vi "Game_Init.vi"(11 "display in":refnum<vi>) -> (0 "error out":errorcluster, 3 "class data out":refnum<class "Game.lvclass">)   [LabVIEW 2010, in "Labricks.lvlib" / "Game.lvclass"]
uses:
  Game.lvclass
  <vilib>/Utility/miscctls.llb/LV3DPointTypeDef.ctl
  BoundingBox_class/BoundingBox.lvclass
  RenderBase/SceneRoot_class/SceneRoot.lvclass
  Game.lvclass/Game.ctl
  Paddle_class/Paddle.lvclass
  Text_class/Text.lvclass
  Ball_class/Ball.lvclass
  RenderBase/SceneObject_class/properties/InitialPosition/SetInitialPosition.vi
  Ball_class/properties/InitialDirection/SetInitialDirection.vi
  RenderBase/Sprite_class/Sprite.lvclass
  RenderBase/SceneObject_class/SceneObject.lvclass
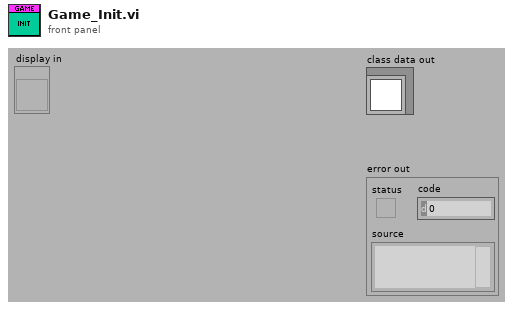
[diagram p1: front panel]
types:
  T1 = typedef "LV3DPointTypeDef.ctl" = cluster{"X":sgl, "Y":sgl, "Z":sgl}
  T2 = cluster{"X":sgl, "Y":sgl, "Width":sgl, "Height":sgl}
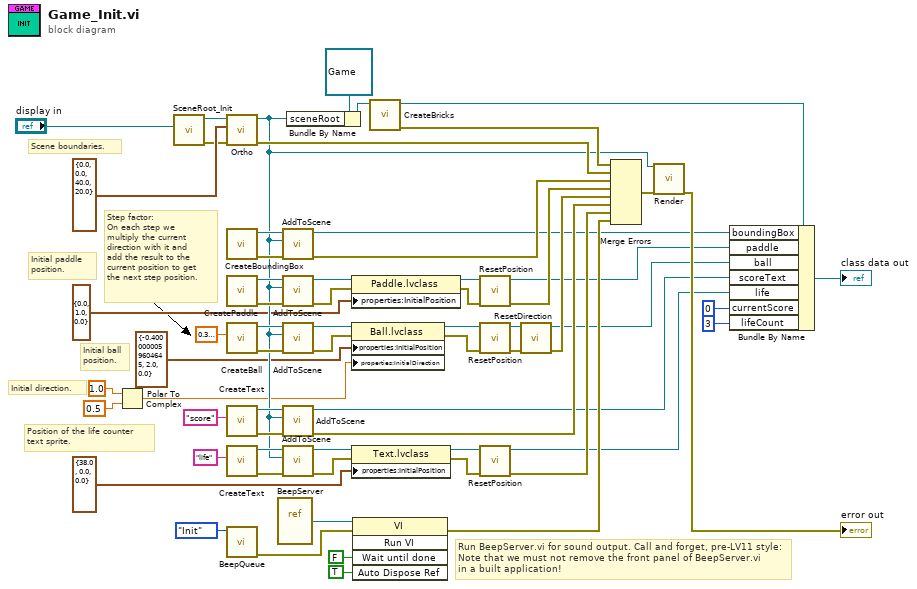
[diagram p0: block diagram]
diagram:
  # "Initial ball\nposition."
  # "Step factor:\nOn each step we\nmultiply the current\ndirection with it and\nadd the result to the\ncurrent position to get\nthe next step position."
  # "Position of the life counter\ntext sprite."
  # "Initial direction."
  # "Initial paddle \nposition."
  # "Scene boundaries."
  # "Run BeepServer.vi for sound output. Call and forget, pre-LV11 style:\nNote that we must not remove the front panel of BeepServer.vi\nin a built application!"
  n1 = Polar To Complex(1:sgl 0.5, 2:sgl 1.0 ("r")) -> (0:w9:csg)
  n2 = call "SceneRoot_Init.vi"("display in"="display in") -> ("error out"=w49:errorcluster, "class data out"=w59:refnum<class "SceneRoot.lvclass">)  [unwired: 9 in]
  n3 = call-dynamic "Ortho.vi"("error in (no error)"=w49, "boundaries in"=T2 {"X"=0.0, "Y"=0.0, "Width"=40.0, "Height"=20.0}, "class data in"=w59) -> ("error out"=w22:errorcluster, "class data out"=w20:refnum<class "SceneRoot.lvclass">)  [unwired: 7 in]
  n4 = call "CreateBoundingBox.vi"() -> ("error out"=w52:errorcluster, "class data out"=w62:refnum<class "BoundingBox.lvclass">)  [unwired: 10 in]
  n5 = call "CreatePaddle.vi"() -> ("error out"=w51:errorcluster, "class data out"=w55:refnum<class "Paddle.lvclass">)  [unwired: 10 in]
  n6 = call "CreateBall.vi"("stepFactor in"=sgl 0.3) -> ("error out"=w50:errorcluster, "class data out"=w56:refnum<class "Ball.lvclass">)  [unwired: 9 in]
  n7 = call "CreateText.vi"("objName in"="score") -> ("error out"=w41:errorcluster, "class data out"=w60:refnum<class "Text.lvclass">)  [unwired: 9 in]
  n8 = call "CreateText.vi"("objName in"="life") -> ("error out"=w37:errorcluster, "class data out"=w36:refnum<class "Text.lvclass">)  [unwired: 9 in]
  n9 = call "BeepQueue.vi"("mode in (Get)"=enum16{"Get", "Init", "Destroy"}."Init") -> ("error out"=w28:errorcluster)  [unwired: 5 in, 1 out]
  n10 = vi-ref "BeepServer.vi"() -> (w29:refnum<vi>)
  n11 = call-dynamic "AddToScene.vi"("error in (no error)"=w52, "sceneRoot in"=w20, "class data in"=w62) -> ("error out"=w43:errorcluster, "class data out"=w5:refnum<class "BoundingBox.lvclass">)  [unwired: 7 in]
  n12 = call-dynamic "AddToScene.vi"("error in (no error)"=w51, "sceneRoot in"=w20, "class data in"=w55) -> ("error out"=w48:errorcluster, "class data out"=w18:refnum<class "Paddle.lvclass">)  [unwired: 7 in]
  n13 = call-dynamic "AddToScene.vi"("error in (no error)"=w50, "sceneRoot in"=w20, "class data in"=w56) -> ("error out"=w45:errorcluster, "class data out"=w46:refnum<class "Ball.lvclass">)  [unwired: 7 in]
  n14 = call-dynamic "AddToScene.vi"("error in (no error)"=w41, "sceneRoot in"=w20, "class data in"=w60) -> ("error out"=w40:errorcluster, "class data out"=w2:refnum<class "Text.lvclass">)  [unwired: 7 in]
  n15 = call-dynamic "AddToScene.vi"("error in (no error)"=w37, "sceneRoot in"=w20, "class data in"=w36) -> ("error out"=w34:errorcluster, "class data out"=w15:refnum<class "Text.lvclass">)  [unwired: 7 in]
  n16 = Bundle By Name(cluster=refnum<class "Game.lvclass"> refnum ("Labricks.lvlib:Game.lvclass"), "sceneRoot"=w20) -> (w32:refnum<class "Game.lvclass">)
  n17 = property class="Paddle.lvclass"(reference=w18, error in=w48, "properties:InitialPosition"=T1 {"X"=0.0, "Y"=1.0, "Z"=0.0} ("targetCoords in")) -> (reference out=w17:refnum<class "Paddle.lvclass">, error out=w19:errorcluster)
  n18 = property class="Ball.lvclass"(reference=w46, error in=w45, "properties:InitialPosition"=T1 {"X"=-0.4, "Y"=2.0, "Z"=0.0} ("InitialPosition"), "properties:InitialDirection"=w9) -> (reference out=w47:refnum<class "Ball.lvclass">, error out=w11:errorcluster)
  n19 = property class="Text.lvclass"(reference=w15, error in=w34, "properties:InitialPosition"=T1 {"X"=38.0, "Y"=0.0, "Z"=0.0} ("targetCoords in")) -> (reference out=w14:refnum<class "Text.lvclass">, error out=w16:errorcluster)
  n20 = invoke class="VI" method="Run VI"(reference=w29, error in=w28, "Wait until done"=FALSE ("Wait Until Done"), "Auto Dispose Ref"=TRUE ("Auto Dispose Reference")) -> (error out=w27:errorcluster)  [unwired: 1 in, 4 out]
  n21 = call "CreateBricks.vi"("class data in"=w32) -> ("error out"=w21:errorcluster, "class data out"=w24:refnum<class "Game.lvclass">)  [unwired: 9 in]
  n22 = call "ResetPosition.vi"("error in"=w19, "class data in"=w17) -> ("error out"=w42:errorcluster, "class data out"=w4:refnum<class "Paddle.lvclass">)  [unwired: 8 in]
  n23 = call "ResetPosition.vi"("error in"=w11, "class data in"=w47) -> ("error out"=w7:errorcluster, "class data out"=w8:refnum<class "Ball.lvclass">)  [unwired: 8 in]
  n24 = call "ResetPosition.vi"("error in"=w16, "class data in"=w14) -> ("error out"=w30:errorcluster, "class data out"=w1:refnum<class "Text.lvclass">)  [unwired: 8 in]
  n25 = call "ResetDirection.vi"("error in"=w7, "class data in"=w8) -> ("error out"=w6:errorcluster, "class data out"=w3:refnum<class "Ball.lvclass">)  [unwired: 8 in]
  n26 = Merge Errors(w21, w22, w43, w42, w6, w40, w30, w27) -> (w44:errorcluster)
  n27 = call-dynamic "Render.vi"("class data in"=w20, "error in (no error)"=w44) -> ("error out"=→"error out":errorcluster)  [unwired: 16 in, 1 out]
  n28 = Bundle By Name(cluster=w24, "boundingBox"=w5, "paddle"=w4, "ball"=w3, "scoreText"=w2, "life"=w1, "currentScore"=0, "lifeCount"=3) -> (→"class data out":refnum<class "Game.lvclass">)
